vi "Josn Test.vi"() -> ()   [LabVIEW 2017]
uses:
  controls/Configuration Details.ctl
panel:
  out "JSON string":string
  out "value 2":string[][](array[string])
  out "value":T1
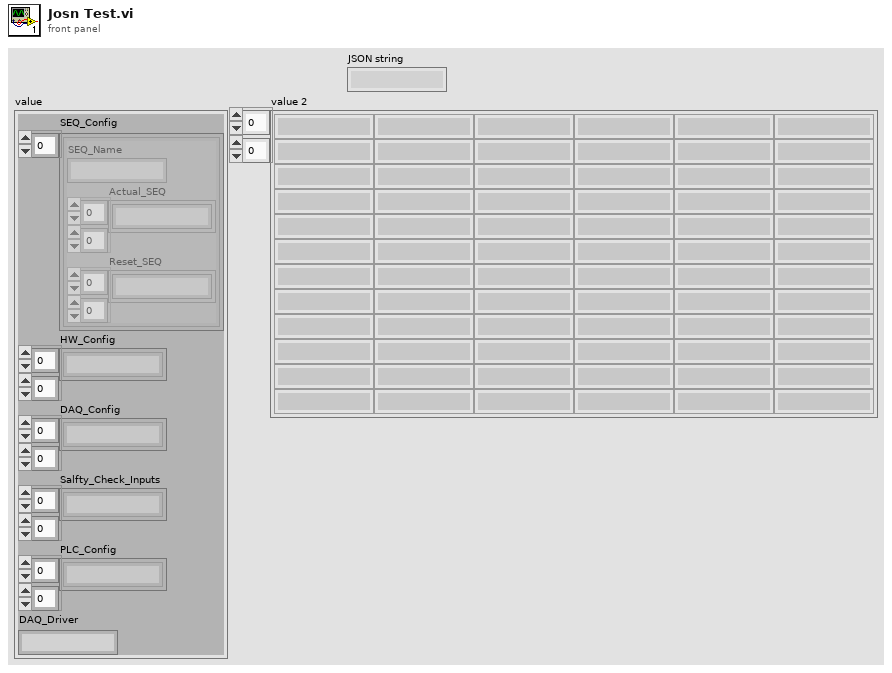
[diagram p1: front panel]
types:
  T1 = typedef "Configuration Details.ctl" = cluster{"SEQ_Config":cluster{"SEQ_Name":string, "Actual_SEQ":string[][], "Reset_SEQ":string[][]}[], "HW_Config":string[][], "DAQ_Config":string[][], "Salfty_Check_Inputs":string[][], "PLC_Config":string[][], "DAQ_Driver":string}
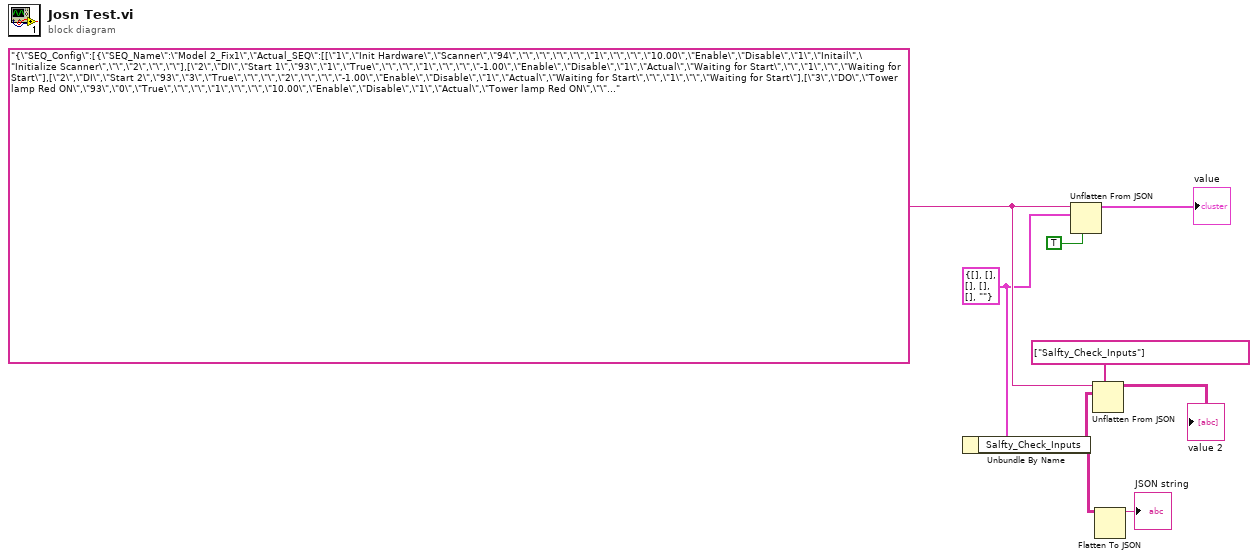
[diagram p0: block diagram]
diagram:
  w5 = T1 {"SEQ_Config"=[], "HW_Config"=[], "DAQ_Config"=[], "Salfty_Check_Inputs"=[], "PLC_Config"=[], "DAQ_Driver"=""} ("Configuration")
  w7 = "{\"SEQ_Config\":[{\"SEQ_Name\":\"Model 2_Fix1\",\"Actual_SEQ\":[[\"1\",\"Init Hardware\",\"Scanner\",\"94\",\"\",\"\",\"\",\"\",\"1\",\"\",\"\",\"10.00\",\"Enable\",\"Disable\",\"1\",\"Initail\",\"Initialize Scanner\",\"\",\"2\",\"\",\"\"],[\"2\",\"DI\",\"Start 1\",\"93\",\"1\",\"True\",\"\",\"\",\"1\",\"\",\"\",\"-1.00\",\"Enable\",\"Disable\",\"1\",\"Actual\",\"Waiting for Start\",\"\",\"1\",\"\",\"Waiting for Start\"],[\"2\",\"DI\",\"Start 2\",\"93\",\"3\",\"True\",\"\",\"\",\"2\",\"\",\"\",\"-1.00\",\"Enable\",\"Disable\",\"1\",\"Actual\",\"Waiting for Start\",\"\",\"1\",\"\",\"Waiting for Start\"],[\"3\",\"DO\",\"Tower lamp Red ON\",\"93\",\"0\",\"True\",\"\",\"\",\"1\",\"\",\"\",\"10.00\",\"Enable\",\"Disable\",\"1\",\"Actual\",\"Tower lamp Red ON\",\"\",\"4\",\"\",\"Tower lamp Red\"],[\"4\",\"Delay\",\"\",\"93\",\"delay\",\"5.00\",\"\",\"\",\"1\",\"\",\"\",\"\",\"Enable\",\"Disable\",\"\",\"Actual\",\"Delay\",\"\",\"5\",\"False\",\"Delay \"],[\"5\",\"DO\",\"Red\",\"93\",\"0\",\"False\",\"\",\"\",\"1\",\"\",\"\",\"10.00\",\"Enable\",\"Disable\",\"0\",\"Actual\",\"Tower Lamp Green ON\",\"\",\"6\",\"\",\"Tower Lamp Green \"],[\"5\",\"DO\",\"Green\",\"93\",\"1\",\"True\",\"\",\"\",\"2\",\"\",\"\",\"10.00\",\"Enable\",\"Disable\",\"0\",\"Actual\",\"Tower Lamp Green ON\",\"\",\"6\",\"\",\"Tower Lamp Green \"],[\"6\",\"Delay\",\"\",\"93\",\"delay\",\"5.00\",\"\",\"\",\"1\",\"\",\"\",\"\",\"Enable\",\"Disable\",\"\",\"Actual\",\"Delay 5s\",\"\",\"2\",\"False\",\"Delay 5s\"]],\"Reset_SEQ\":[[]]}],\"HW_Config\":[[\"94\",\"Scanner\",\"Cognex Fixed Serial\",\"IP Address=COM98,|Baud rate=115200.000000,|Timeout (10sec)=10.000000,\"]],\"DAQ_Config\":[[\"Estop\",\"DI,1,0\",\"DI\"],[\"Start 1\",\"DI,1,1\",\"DI\"],[\"Reset\",\"DI,1,2\",\"DI\"],[\"Start 2\",\"DI,1,3\",\"DI\"],[\"Input Type\",\"10106\",\"\"],[\"Sample Mode\",\"10123\",\"\"],[\"No. of samples\",\"0.000000\",\"\"],[\"Minimum Value\",\"0.000000\",\"\"],[\"Maximum Value\",\"0.000000\",\"\"],[\"Sampling Rate\",\"0.000000\",\"\"],[\"Com Port\",\"1.000000\",\"\"],[\"LIGHT CURTAIN FB\",\"DI,1,4\",\"DI\"],[\"PRESSURE SWITCH FB\",\"DI,1,5\",\"DI\"],[\"CLAMP 1\",\"DI,1,6\",\"DI\"],[\"UNCLAMP 1\",\"DI,1,7\",\"DI\"],[\"CLAMP 2\",\"DI,1,8\",\"DI\"],[\"UNCLAMP 2\",\"DI,1,9\",\"DI\"],[\"Tower lamp Red\",\"DO,3,0\",\"DO\"],[\"Tower lamp Green\",\"DO,3,1\",\"DO\"],[\"Tower lamp Yellow\",\"DO,3,2\",\"DO\"],[\"Tower lamp Buzzer\",\"DO,3,3\",\"DO\"],[\"LINEAR CYL @ HOME\",\"DI,1,10\",\"DI\"],[\"LINEAR CYL @ TEST\",\"DI,1,11\",\"DI\"],[\"SHUTTER CYL @ HOME\",\"DI,1,12\",\"DI\"],[\"SHUTTER CYL @ TEST\",\"DI,1,13\",\"DI\"],[\"CAMERA CYL @ HOME\",\"DI,1,14\",\"DI\"],[\"CAMERA CYL @ TEST\",\"DI,1,15\",\"DI\"],[\"AIR BOOTH SENSOR\",\"DI,2,0\",\"DI\"],[\"PART PRESENCE\",\"DI,2,1\",\"DI\"],[\"PEEL OFF SENSOR\",\"DI,2,2\",\"DI\"],[\"DIFFUSER SENSOR\",\"DI,2,3\",\"DI\"],[\"Clamp 1\",\"DO,3,4\",\"DO\"],[\"UNClamp 1\",\"DO,3,5\",\"DO\"],[\"LINEAR CYL @ HOME\",\"DO,3,6\",\"DO\"],[\"LINEAR CYL @ TEST\",\"DO,3,7\",\"DO\"],[\"SHUTTER CYL @ HOME\",\"DO,3,8\",\"DO\"],[\"SHUTTER CYL @ TEST\",\"DO,3,9\",\"DO\"],[\"CAMERA CYL @ HOME\",\"DO,3,10\",\"DO\"],[\"CAMERA CYL @ TEST\",\"DO,3,12\",\"DO\"],[\"AIR BOOTH ON/OFF\",\"DO,5,12\",\"DO\"],[\"SUCTION ON/OFF\",\"DO,3,13\",\"DO\"],[\"MAIN AIR ON/OFF\",\"DO,3,14\",\"DO\"],[\"CAMERA 1 LIGHT ON/OFF\",\"DO,3,15\",\"DO\"],[\"CAMERA 2 LIGHT ON/OFF\",\"DO,4,0\",\"DO\"]],\"Salfty_Check_Inputs\":[[]],\"PLC_Config\":[[]],\"DAQ_Driver\":\"ICP con\"}" ("JSON string")
  n1 = Unbundle By Name(w5) -> ("Salfty_Check_Inputs"=w2:string[][])
  n2 = Unflatten From JSON(JSON string=w7, type and defaults=w5, default null elements? (F)=TRUE) -> (value=→"value":T1)  [unwired: 4 in, 1 out]
  n3 = Unflatten From JSON(path=string[] ["Salfty_Check_Inputs"], JSON string=w7, type and defaults=w2) -> (value=→"value 2":string[][])  [unwired: 4 in, 1 out]
  n4 = Flatten To JSON(anything=w2) -> (JSON string=→"JSON string":string)  [unwired: 2 in, 1 out]
